vi "Google - Get Data (for stock ticker).vi"(0 "Symbol":string, 3 "error in":errorcluster) -> (6 "Stock Data":T1, 9 "error out":errorcluster)   [LabVIEW 2011]
doc: "Get the symbol data from Google Finance.\n\nInputs:\n Symbol: Stock ticker symbol.\n Error in: Describes error conditions that occur before this node runs. This input provides standard error in functionality.\n\nOutputs:\n Stock Data: Parsed Stock Data\n Symbol\n Name\n Price\n Change\n Change %\n Volume: N/A\n Error out: Contains error information. This output provides standard error out functionality."
uses:
  Stock Data Control.ctl
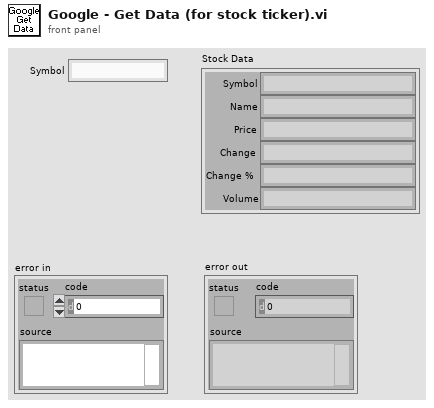
[diagram p1: front panel]
types:
  T1 = typedef "Stock Data Control.ctl" = cluster{"Symbol":string, "Name":string, "Price":string, "Change":string, "Change %":string, "Volume":string}
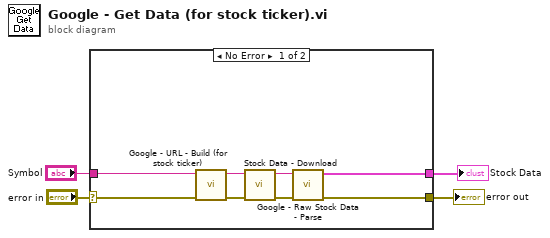
[diagram p0: block diagram]
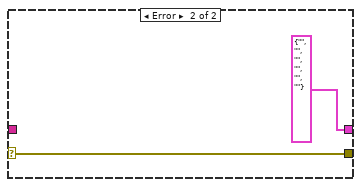
[diagram p2: hidden frame]
diagram:
  n1 = case shown="No Error" "error in" {
    selector: "error in" -> [w8 w14]
    tunnel: [w7 w14] -> w4
    tunnel: "Symbol" -> [w6 _]
    tunnel: [w5 T1 {"Symbol"="", "Name"="", "Price"="", "Change"="", "Change %"="", "Volume"=""} ("Stock Data")] -> w1
    frame No Error {
      n2 = call "Google - URL - Build (for stock ticker).vi"("Symbol"=w6, "error in"=w8) -> ("URL"=w11:string, "error out"=w10:errorcluster)  [unwired: 6 in]
      n3 = call "Stock Data - Download.vi"("error in"=w10, "URL"=w11) -> ("error out"=w9:errorcluster, "Raw Stock Data"=w12:string)  [unwired: 7 in, 1 out]
      n4 = call "Google - Raw Stock Data - Parse.vi"("Raw Stock Data"=w12, "error in"=w9) -> ("Stock Data"=w5:T1, "error out"=w7:errorcluster)  [unwired: 7 in]
    }
    frame Error {
    }
  }
  "error out" <- w4
  "Stock Data" <- w1
